vi "potenciometro_while.vi"() -> ()   [LabVIEW 2023]
uses:
  <vilib>/MakerHub/LINX/Public/Peripherals/Analog/Analog Read 1 Chan.vi
  <vilib>/MakerHub/LINX/Public/Peripherals/Analog/Analog Read N Chans.vi
  <vilib>/MakerHub/LINX/Private/Local IO/LinxAnalogRead.vi
  <vilib>/MakerHub/LINX/Public/Utilities/Check Channel.vi
  <vilib>/MakerHub/LINX/Public/Utilities/Open Serial.vi
  <vilib>/MakerHub/LINX/Private/Utilties/Generate Error.vi
  <vilib>/MakerHub/LINX/LMH-LINX.lvlib
panel:
  out "Loop Rate (Hz)":u32=5
  out "NS":dbl=51.0
  in  "tsim":dbl=10.0
  out "Ts":dbl=0.2
  in  "fs":dbl=5.0
  out "IT":i32=50
  out "Chart":dbl(graph)=0.869140625
  # "CON ESTO SE GENERA MI ARCHIVO data-pot.lvm"
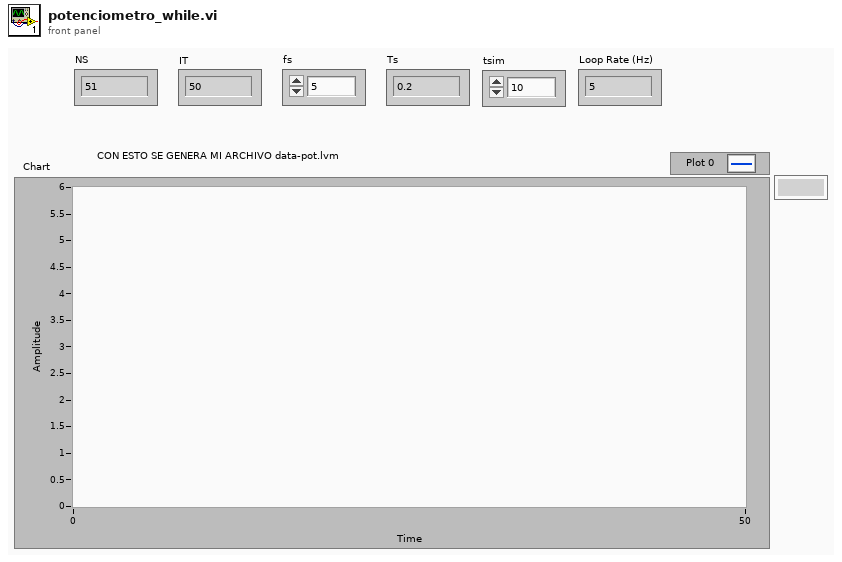
[diagram p1: front panel]
types:
  T1 = typedef "LMH-LINX.lvlib/LINX Ref.ctl" = cluster{"IO":T2, "Interface":T3, "LINX Device Config":T4}
  T2 = typedef "LMH-LINX.lvlib/Platform.ctl" = enum16{"Remote", "Local"}
  T3 = typedef "LMH-LINX.lvlib/Interface.ctl" = enum16{"Serial", "TCP"}
  T4 = typedef "LMH-LINX.lvlib/Device.lvlib/LINX Device Config.ctl" = cluster{"Interface":T3, "COM Port":refnum<visa-resource-name>, "TCP Configuration":T5, "Device Family":u8, "Device ID":u8, "Device Name":string, "TCP Ref":refnum<k5>, "Channels":T6}
  T5 = typedef "LMH-LINX.lvlib/Device.lvlib/TCP Config.ctl" = cluster{"IP Address":string, "Port":u16}
  T6 = typedef "LMH-LINX.lvlib/Channels.ctl" = cluster{"DI":u8[], "DO":u8[], "AI":u8[], "AO":u8[], "PWM":u8[], "QE":u8[], "UART":u8[], "I2C 2":u8[], "SPI":u8[], "CAN":u8[], "Servo":u8[], "AI Ref (V)":dbl, "AI Resolution (Bits)":u8, "AO Ref (V)":dbl, "AO Resolution (Bits)":u8}
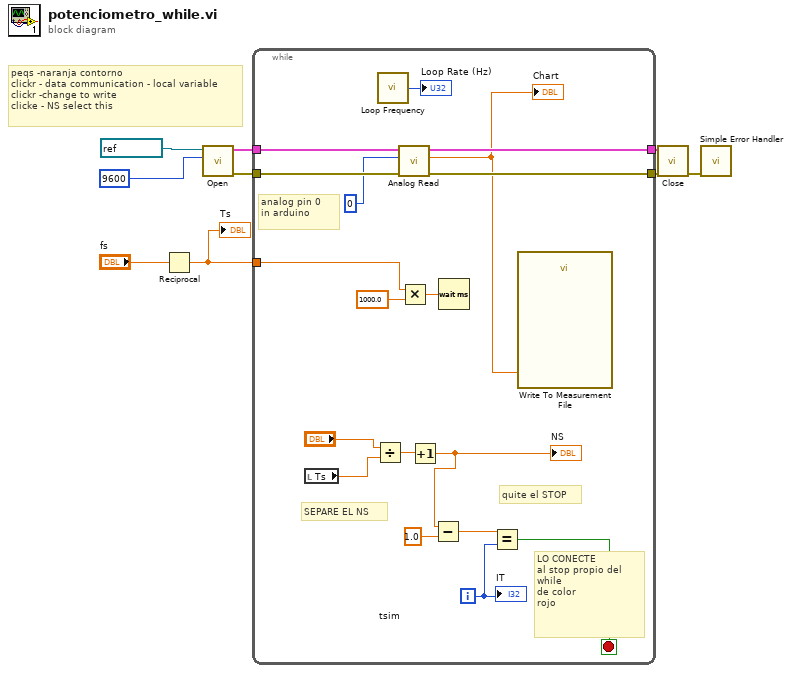
[diagram p0: block diagram]
diagram:
  # "peqs -naranja contorno \nclickr - data communication - local variable\nclickr -change to write\nclicke - NS select this"
  n1 = Reciprocal(x="fs") -> (1/x=w8:dbl)
  "Ts" <- w8
  n2 = call-poly <vilib>:"Open.vi"("Baud Rate Override"=u32 9600, "Serial Port"=refnum<visa-resource-name> "COM7") -> ("Error Out"=w6:errorcluster, "LINX Resource"=w7:T1)  [unwired: 7 in, 1 out]
  n3 = while {
    tunnel: w8 -> [w22]
    tunnel: w7 -> [w21]
    tunnel: w6 -> [w20]
    tunnel: [w19] -> w5
    tunnel: [w18] -> w4
    i -> [w25]
    stop <- w10 stop-if-true
    # "LO CONECTE\nal stop propio del\nwhile\nde color \nrojo"
    # "SEPARE EL NS"
    # "quite el STOP"
    # "analog pin 0 \nin arduino"
    n4 = local read "Ts"() -> (w14:dbl)
    n5 = Divide(x="tsim", y=w14) -> (x/y=w13:dbl)
    n6 = call <vilib>:"Loop Frequency.vi"() -> ("Loop Rate (Hz)"=→"Loop Rate (Hz)":u32)
    n7 = call-poly <vilib>:"Analog Read.vi"("Error In"=w20, "Analog Channel"=u8 0, "LINX Resource"=w21) -> ("Error Out"=w19:errorcluster, "Voltage"=w17:dbl, "LINX Resource"=w18:T1)  [unwired: 5 in, 1 out]
    "Chart" <- w17
    n8 = Multiply(x=w22, y=1000.0) -> (x*y=w27:dbl)
    n9 = Increment(x=w13) -> (x+1=w11:dbl)
    "NS" <- w11
    n10 = Subtract(x=w11, y=1.0) -> (x-y=w23:dbl)
    n11 = Wait (ms)(milliseconds to wait=w27) -> ()  [unwired: 1 out]
    n12 = Equal?(x=w23, y=w25) -> (x = y?=w10:bool)
    n13 = call "Write To Measurement File"("Signals"=w17) -> ()  [unwired: 16 in, 3 out]
    "IT" <- w25
  }
  n14 = call <vilib>:"Close.vi"("Error In"=w5, "LINX Resource"=w4) -> ("Error Out"=w1:errorcluster)  [unwired: 9 in]
  n15 = call <vilib>:"Simple Error Handler.vi"("error in (no error)"=w1) -> ()  [unwired: 4 in, 5 out]
